vi "pBot_waitForMoveFinish.vi"(10 "disconnectPBot_Event":refnum<user-event>, 11 "pBot_VISA":refnum<visa-resource-name>) -> (0 "errorOut":errorcluster, 3 "moveFinished?":bool)   [LabVIEW 2015]
uses:
  approxEqualvecDBL.vi
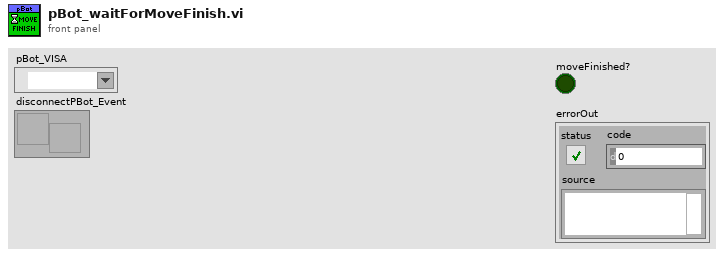
[diagram p1: front panel]
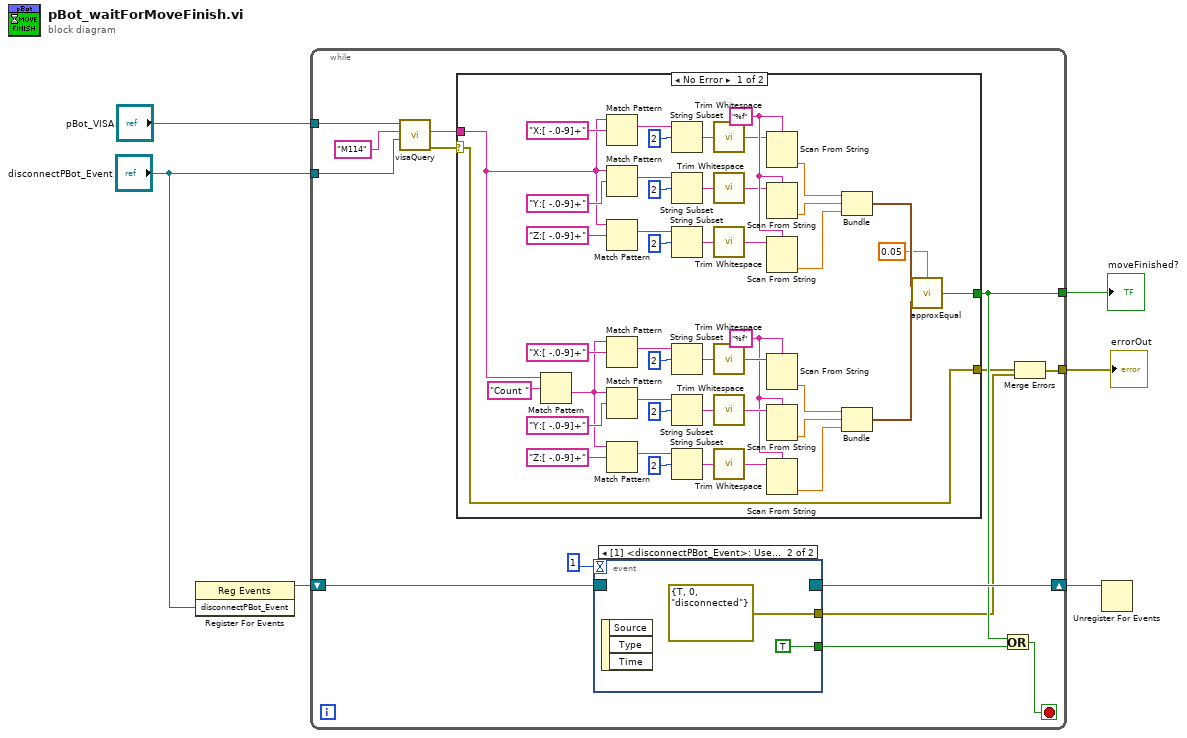
[diagram p0: block diagram]
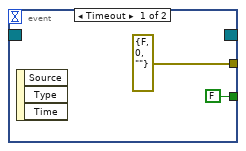
[diagram p2: hidden frame]
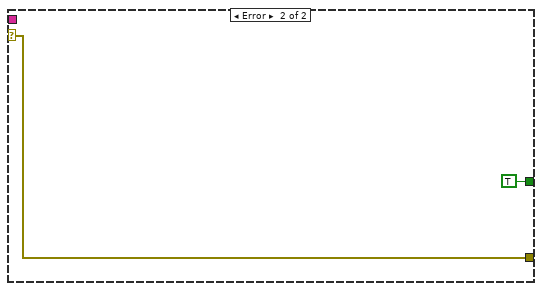
[diagram p3: hidden frame]
diagram:
  n1 = register-events("disconnectPBot_Event") -> (reference out=w4:refnum<event-registration>)  [unwired: 2 in, 1 out]
  n2 = while {
    tunnel: "pBot_VISA" -> [w18]
    tunnel: "disconnectPBot_Event" -> [w16]
    shift-right: [w11] -> w1
    shift-left: w4 -> [w14]
    tunnel: [w10] -> w2
    tunnel: [w9] -> w3
    stop <- w12 stop-if-true
    n3 = call "visaQuery.vi"("disconnectPBot_Event"=w16, "stringToWrite"="M114", "VISA resource name"=w18) -> ("error Out"=w17:errorcluster, "String"=w20:string)  [unwired: 6 in, 1 out]
    n4 = case shown="No Error" w17 {
      selector: w17 -> [w25 w71]
      tunnel: w20 -> [w37 _]
      tunnel: [w26 TRUE ("approximatelyEqual?")] -> w10
      tunnel: [w25 w71] -> w8
      frame No Error {
        w39 = "%f" ("format string")
        w70 = "%f" ("format string")
        n5 = Match Pattern(string=w37, regular expression="Count ") -> (after substring=w36:string)  [unwired: 1 in, 3 out]
        n6 = Match Pattern(string=w37, regular expression="X:[ -.0-9]+") -> (match substring=w58:string)  [unwired: 1 in, 3 out]
        n7 = Match Pattern(string=w37, regular expression="Y:[ -.0-9]+") -> (match substring=w63:string)  [unwired: 1 in, 3 out]
        n8 = Match Pattern(string=w37, regular expression="Z:[ -.0-9]+") -> (match substring=w62:string)  [unwired: 1 in, 3 out]
        n9 = Match Pattern(string=w36, regular expression="X:[ -.0-9]+") -> (match substring=w51:string)  [unwired: 1 in, 3 out]
        n10 = Match Pattern(string=w36, regular expression="Y:[ -.0-9]+") -> (match substring=w46:string)  [unwired: 1 in, 3 out]
        n11 = Match Pattern(string=w36, regular expression="Z:[ -.0-9]+") -> (match substring=w47:string)  [unwired: 1 in, 3 out]
        n12 = String Subset(string=w58, offset (0)=2) -> (substring=w64:string)  [unwired: 1 in]
        n13 = String Subset(string=w63, offset (0)=2) -> (substring=w66:string)  [unwired: 1 in]
        n14 = String Subset(string=w62, offset (0)=2) -> (substring=w65:string)  [unwired: 1 in]
        n15 = String Subset(string=w51, offset (0)=2) -> (substring=w45:string)  [unwired: 1 in]
        n16 = String Subset(string=w46, offset (0)=2) -> (substring=w43:string)  [unwired: 1 in]
        n17 = String Subset(string=w47, offset (0)=2) -> (substring=w44:string)  [unwired: 1 in]
        n18 = call <vilib>:"Trim Whitespace.vi"("string"=w64) -> ("trimmed string"=w67:string)  [unwired: 1 in]
        n19 = call <vilib>:"Trim Whitespace.vi"("string"=w66) -> ("trimmed string"=w69:string)  [unwired: 1 in]
        n20 = call <vilib>:"Trim Whitespace.vi"("string"=w65) -> ("trimmed string"=w68:string)  [unwired: 1 in]
        n21 = call <vilib>:"Trim Whitespace.vi"("string"=w45) -> ("trimmed string"=w42:string)  [unwired: 1 in]
        n22 = call <vilib>:"Trim Whitespace.vi"("string"=w43) -> ("trimmed string"=w40:string)  [unwired: 1 in]
        n23 = call <vilib>:"Trim Whitespace.vi"("string"=w44) -> ("trimmed string"=w41:string)  [unwired: 1 in]
        n24 = Scan From String(format string=w70, input string=w67) -> (output 1=w35:dbl)  [unwired: 3 in, 3 out]
        n25 = Scan From String(format string=w70, input string=w69) -> (output 1=w34:dbl)  [unwired: 3 in, 3 out]
        n26 = Scan From String(format string=w70, input string=w68) -> (output 1=w33:dbl)  [unwired: 3 in, 3 out]
        n27 = Scan From String(format string=w39, input string=w42) -> (output 1=w32:dbl)  [unwired: 3 in, 3 out]
        n28 = Scan From String(format string=w39, input string=w40) -> (output 1=w31:dbl)  [unwired: 3 in, 3 out]
        n29 = Scan From String(format string=w39, input string=w41) -> (output 1=w30:dbl)  [unwired: 3 in, 3 out]
        n30 = Bundle(w35, w34, w33) -> (w29:cluster{dbl, dbl, dbl})  [unwired: 1 in]
        n31 = Bundle(w32, w31, w30) -> (w28:cluster{dbl, dbl, dbl})  [unwired: 1 in]
        n32 = call-poly "approxEqual.vi"("tol (1E-5)"=0.05, "in2"=w28, "in1"=w29) -> ("approximatelyEqual?"=w26:bool)
      }
      frame Error {
      }
    }
    n33 = event shown="[1] <disconnectPBot_Event>: User Event" {
      selector: w14 -> [_ _]
      dyn-events: [_ _] -> w11
      timeout: 1 -> [_ _]
      tunnel: [FALSE TRUE] -> w13
      tunnel: [errorcluster {"status"=FALSE, "code"=0, "source"=""} ("error constant") errorcluster {"status"=TRUE, "code"=0, "source"="disconnected"} ("error constant")] -> w7
      event Timeout {
        n34 = event-data() -> ()  [unwired: 1 in, 3 out]
      }
      event User Event {
        n35 = event-data() -> ()  [unwired: 1 in, 3 out]
      }
    }
    n36 = Or(x=w10, y=w13) -> (x .or. y?=w12:bool)
    n37 = Merge Errors(w8, w7) -> (w9:errorcluster)
  }
  "errorOut" <- w3
  "moveFinished?" <- w2
  n38 = Unregister For Events(event registration refnum=w1) -> ()  [unwired: 1 in, 1 out]
